vi "fgv_Live Imaging status.vi"(8 "error in (no error)":errorcluster, 9 "Function":T1, 11 "Live Imaging?":bool) -> (0 "error out":errorcluster, 3 "Live Imaging?":bool)   [LabVIEW 2020]
uses:
  Typedefs/Read Write Enum.ctl
  General Globals.vi
panel:
  # "SUBROUTINE"
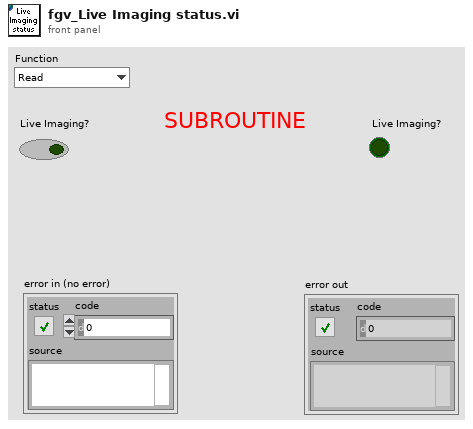
[diagram p1: front panel]
types:
  T1 = typedef "Read Write Enum.ctl" = enum16{"Read", "Write"}
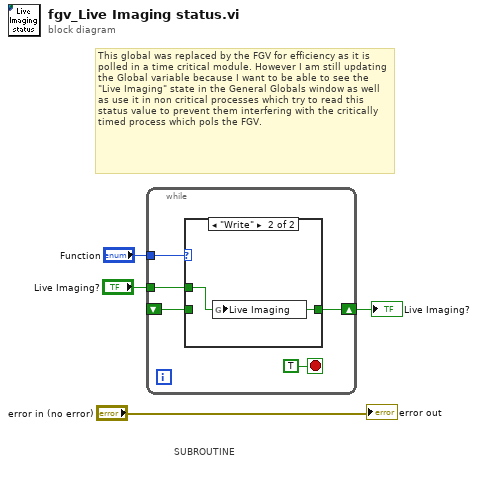
[diagram p0: block diagram]
diagram:
  # "This global was replaced by the FGV for efficiency as it is polled in a time critical module. However I am still updating the Global variable because I want to be able to see the \"Live Imaging\" state in the General Globals window as well as use it in non critical processes which try to read this status value to prevent them interfering with the critically timed process which pols the FGV."
  # "SUBROUTINE"
  n1 = while {
    tunnel: "Function" -> [w8]
    tunnel: "Live Imaging?" -> [w7]
    shift-right: [w6] -> w2
    shift-left: _ -> [w5]
    stop <- TRUE stop-if-true
    n2 = case shown="\"Write\"" w8 {
      tunnel: w7 -> [_ w11]
      tunnel: [w10 w11] -> w6
      tunnel: w5 -> [w10 _]
      frame "Read", Default {
      }
      frame "Write" {
        n3 = global write "General Globals.vi" "Live Imaging"(w11) -> ()
      }
    }
  }
  "Live Imaging?" <- w2
  "error out" <- "error in (no error)"
